vi "GV-ZoomVerticalDrag.vi"(6 "Y":dbl, 7 "Gviewer in":refnum<class "Gviewer.lvclass">, 8 "error in (no error)":errorcluster, 10 "Coords":T1, 11 "pict in":picture) -> (0 "error out":errorcluster, 3 "pict out":picture)   [LabVIEW 2020, in "Sgraph_lib_V1.lvlib" / "Gviewer.lvclass"]
doc: "Andre Koelewijn, 8 May 2021\n\nDraw the zoom Vertical Zoon area"
uses:
  Gviewer.lvclass
  <vilib>/Utility/miscctls.llb/LVPoint32TypeDef.ctl
  Gviewer.lvclass/Gviewer.ctl
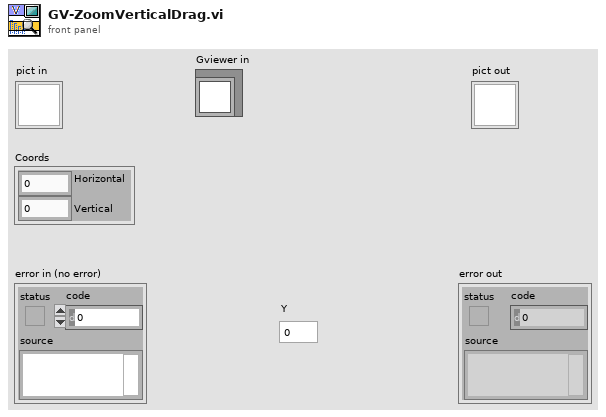
[diagram p1: front panel]
types:
  T1 = typedef "LVPoint32TypeDef.ctl" = cluster{"Horizontal":i32, "Vertical":i32}
  T2 = cluster{"Width":i16, "Style":enum32{"Solid", "Dash", "Dot", "DashDot", "DashDotDot"}}
  T3 = cluster{"left":i16, "top":i16, "right":i16, "bottom":i16}
  T4 = cluster{"horizontal":enum16{"left", "center", "right"}, "vertical":enum16{"top", "center", "bottom"}}
  T5 = typedef "Sgraph_lib_V1.lvlib/Gviewer.lvclass/Typedef_SelProperties.ctl" = cluster{"Color":u32, "LineType":T6, "max":dbl, "min":dbl}
  T6 = typedef "Sgraph_lib_V1.lvlib/Gviewer.lvclass/Typedef_LineType.ctl" = enum16{"num_bare", "num_MinMax_Area", "num_MinMax_Lines", "num_MinMax_Forfor", "num_Max_Area", "num_Max_Line", "num_Max_Forfor", "num_Min_Area", "num_Min_Line", "num_Min_Fosfor", "Boolean_Line_01", "Boolean_Area_01", "Boolean_Fosfor_01", "Boolean_Line_TF", "Boolean_Area_TF", "Boolean_Fosfor_TF", "Boolean_OnOff_Line", "Boolean_OnOff_Area", "Boolean_OnOff_Fosfor", "Boolean_spare", "StringEvent_Line", "StringEvent_TimeLine"}
  T7 = typedef "LVRectTypeDef.ctl" = cluster{"Left":i16, "Top":i16, "Right":i16, "Bottom":i16}
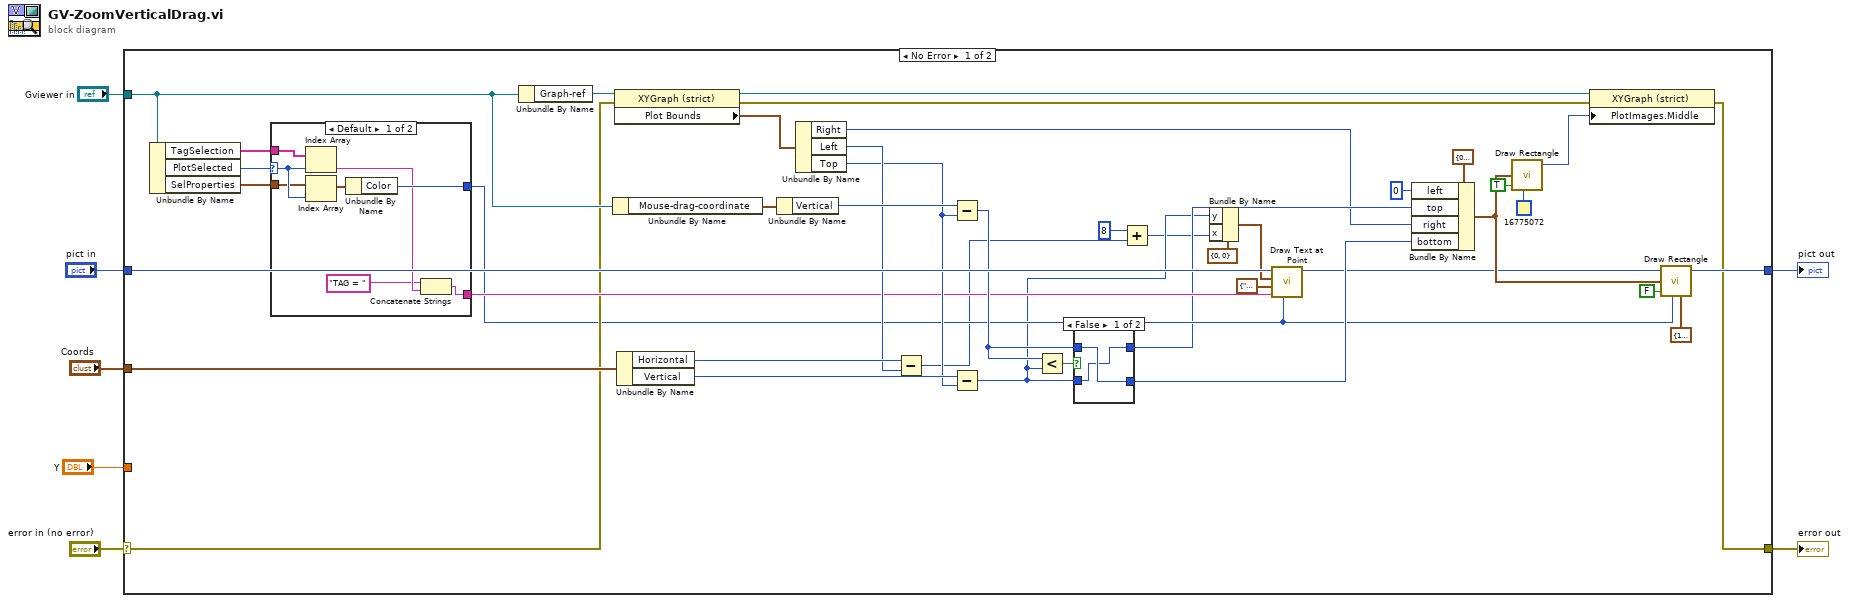
[diagram p0: block diagram]
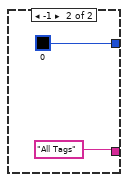
[diagram p2: hidden frame]
diagram:
  n1 = case shown="No Error" "error in (no error)" {
    selector: "error in (no error)" -> [w23 w65]
    tunnel: [w21 w65] -> w6
    tunnel: "pict in" -> [w48 w64]
    tunnel: [w32 w64] -> w4
    tunnel: "Coords" -> [w47 _]
    tunnel: "Gviewer in" -> [w28 _]
    tunnel: "Y" -> [_ _]
    frame No Error {
      n2 = Unbundle By Name(w28) -> ("TagSelection"=w30:string[], "PlotSelected"=w27:i32, "SelProperties"=w29:T5[])
      n3 = case shown="Default" w27 {
        selector: w27 -> [w54 _]
        tunnel: w30 -> [w57 _]
        tunnel: [w52 "All Tags"] -> w26
        tunnel: w29 -> [w51 _]
        tunnel: [w55 u32 0 ("Color")] -> w18
        frame Default {
          n4 = Index Array(array=w57, index=w54) -> (element=w53:string)
          n5 = Index Array(array=w51, index=w54) -> (element=w56:T5)
          n6 = Unbundle By Name(w56) -> ("Color"=w55:u32)
          n7 = Concatenate Strings("TAG = ", w53) -> (w52:string)
        }
        frame -1 {
        }
      }
      n8 = Unbundle By Name(w28) -> ("Graph-ref"=w42:refnum<vi>)
      n9 = Unbundle By Name(w28) -> ("Mouse-drag-coordinate"=w22:T1)
      n10 = property class="XYGraph (strict)"(reference=w42, error in=w23) -> (reference out=w14:refnum<vi>, error out=w13:errorcluster, "Plot Bounds"=w41:T7)
      n11 = Unbundle By Name(w47) -> ("Horizontal"=w39:i32, "Vertical"=w37:i32)
      n12 = Unbundle By Name(w22) -> ("Vertical"=w40:i32)
      n13 = Unbundle By Name(w41) -> ("Right"=w12:i16, "Left"=w38:i16, "Top"=w36:i16)
      n14 = Subtract(x=w39, y=w38) -> (x-y=w10:i32)
      n15 = Subtract(x=w40, y=w36) -> (x-y=w35:i32)
      n16 = Subtract(x=w37, y=w36) -> (x-y=w11:i32)
      n17 = Less?(x=w35, y=w11) -> (x < y?=w34:bool)
      n18 = case shown="False" w34 {
        tunnel: w35 -> [w61 w63]
        tunnel: [w60 w63] -> w16
        tunnel: [w61 w62] -> w19
        tunnel: w11 -> [w60 w62]
        frame False {
        }
        frame True {
        }
      }
      n19 = Add(x=8, y=w10) -> (x+y=w8:i32)
      n20 = Bundle By Name(cluster=cluster{"x":i16, "y":i16} {"x"=0, "y"=0} ("origin"), "y"=w11, "x"=w8) -> (w24:cluster{"x":i16, "y":i16})
      n21 = call <vilib>:"Draw Text at Point.vi"("text color(black)"=w18, "text"=w26, "alignment(left, top)"=T4 {"horizontal"=enum."center", "vertical"=enum."bottom"}, "origin"=w24, "picture"=w48) -> ("new picture"=w17:picture)  [unwired: 5 in, 1 out]
      n22 = Bundle By Name(cluster=T3 {"left"=0, "top"=0, "right"=0, "bottom"=0} ("rect"), "left"=i16 0, "top"=w16, "right"=w12, "bottom"=w19) -> (w20:T3)
      n23 = call <vilib>:"Draw Rectangle.vi"("rect"=w20, "fill?(F)"=TRUE, "color(black)"=u32 16775072) -> ("new picture"=w46:picture)  [unwired: 6 in]
      n24 = property class="XYGraph (strict)"(reference=w14, error in=w13, "PlotImages.Middle"=w46) -> (error out=w21:errorcluster)  [unwired: 1 out]
      n25 = call <vilib>:"Draw Rectangle.vi"("picture"=w17, "rect"=w20, "fill?(F)"=FALSE, "color(black)"=w18, "pen"=T2 {"Width"=1, "Style"=enum."Dot"}) -> ("new picture"=w32:picture)  [unwired: 4 in]
    }
    frame Error {
    }
  }
  "error out" <- w6
  "pict out" <- w4
